vi "Lookup Implementation.vi"(8 "error in (no error)":errorcluster, 10 "Implementation Tag":string, 11 "Dynamic Dispatch VI Type in":refnum<class "Dynamic Dispatch VI Type.lvclass">) -> (0 "error out":errorcluster, 2 "Found?":bool, 3 "Dynamic Dispatch VI Type out":refnum<class "Dynamic Dispatch VI Type.lvclass">)   [LabVIEW 2020, in "Peek Window.lvlib" / "Dynamic Dispatch VI Type.lvclass"]
uses:
  Dynamic Dispatch VI Type.lvclass
  D:/Code/VI-Peek/source/Peek Window/VI Types/Standard VI Type/Standard VI Type.lvclass
  Dynamic Dispatch VI Type.lvclass/Dynamic Dispatch VI Type.ctl
  Standard VI Type/Standard VI Type.lvclass/Standard VI Type.ctl
  Standard VI Type/Read VI Refnum.vi
  Standard VI Type/Read Full Qualified Name.vi
  Standard VI Type/Write VI Refnum.vi
  Standard VI Type/Write Full Qualified Name.vi
  Implementation VI Type/Implementation VI Type.lvclass
  <vilib>/Utility/error.llb/Error Cluster From Error Code.vi
  <vilib>/ErrorRing/Error Ring.xnode
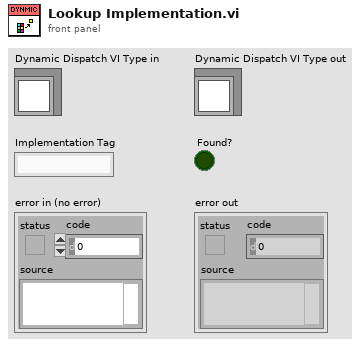
[diagram p1: front panel]
types:
  T1 = map{string, refnum<class "Implementation VI Type.lvclass">}
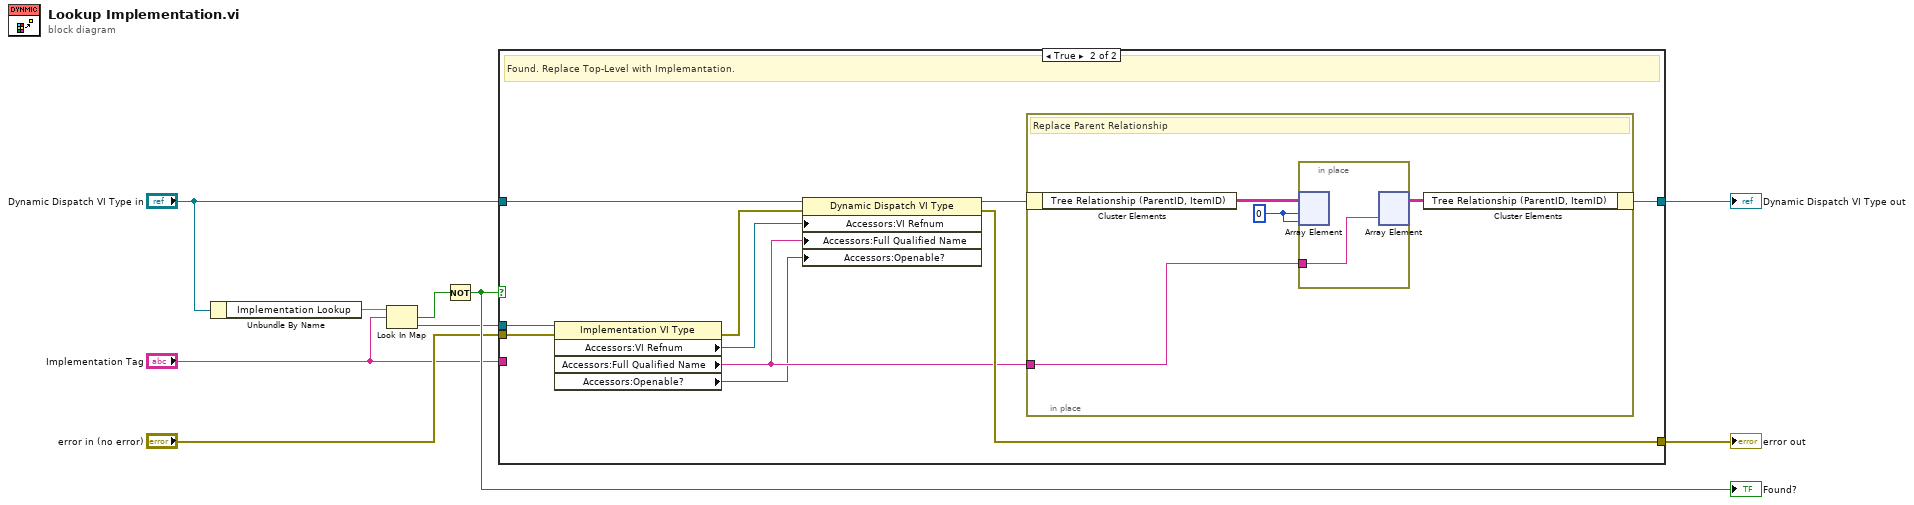
[diagram p0: block diagram]
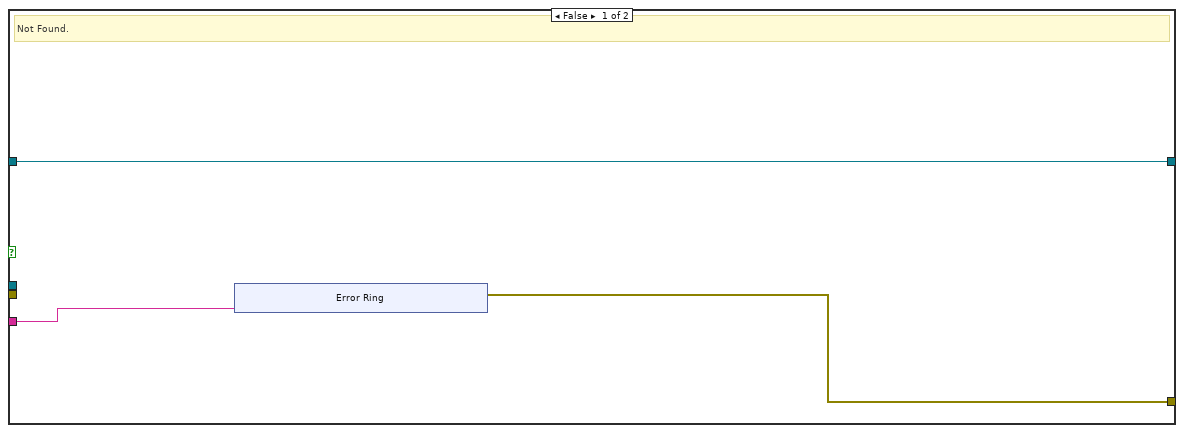
[diagram p2: hidden frame]
diagram:
  n1 = Unbundle By Name("Dynamic Dispatch VI Type in") -> ("Implementation Lookup"=w7:T1)
  n2 = Look In Map(map=w7, key="Implementation Tag") -> (key not found?=w8:bool, value=w3:refnum<class "Implementation VI Type.lvclass">)  [unwired: 1 in]
  n3 = Not(x=w8) -> (.not. x?=w4:bool)
  "Found?" <- w4
  n4 = case shown="True" w4 {
    tunnel: "Dynamic Dispatch VI Type in" -> [w12 w29]
    tunnel: [w12 w22] -> w6
    tunnel: [w10 w28] -> w5
    tunnel: w3 -> [_ w27]
    tunnel: "error in (no error)" -> [_ w26]
    tunnel: "Implementation Tag" -> [w11 _]
    frame False {
      # "Not Found."
      n5 = xnode "Error Ring"("parameter 0"=w11) -> ("error out"=w10:errorcluster)
    }
    frame True {
      # "Found. Replace Top-Level with Implemantation."
      n6 = property class="Implementation VI Type"(reference=w27, error in=w26) -> (error out=w25:errorcluster, "Accessors:VI Refnum"=w24:refnum<vi>, "Accessors:Full Qualified Name"=w21:string, "Accessors:Openable?"=w20:bool)  [unwired: 1 out]
      n7 = property class="Dynamic Dispatch VI Type"(reference=w29, error in=w25, "Accessors:VI Refnum"=w24, "Accessors:Full Qualified Name"=w21, "Accessors:Openable?"=w20) -> (reference out=w23:refnum<class "Dynamic Dispatch VI Type.lvclass">, error out=w28:errorcluster)
      n8 = in-place {
        in-place-border: w21 -> [w31]
        w32 = 0
        # "Replace Parent Relationship"
        n9 = in-place-cluster #1(w23) -> ("Tree Relationship (ParentID, ItemID)"=w33:string[][])
        n10 = in-place {
          in-place-border: w31 -> [w34]
          n11 = in-place-array #2(w33, w32, w32) -> ()  [unwired: 1 out]
          n12 = in-place-array #2(w34) -> (w30:string[][])  [unwired: 2 out]
        }
        n13 = in-place-cluster #1("Tree Relationship (ParentID, ItemID)"=w30) -> (w22:refnum<class "Dynamic Dispatch VI Type.lvclass">)
      }
    }
  }
  "error out" <- w5
  "Dynamic Dispatch VI Type out" <- w6
